vi "Initialize position.vi"(8 "error in (no error)":errorcluster) -> (0 "error out":errorcluster, 3 "Position out":refnum<class "Position.lvclass">)   [LabVIEW 2016, in "Chesslib.lvlib" / "Position.lvclass"]
uses:
  Position.lvclass
  typedef/Color.ctl
  typedef/Square.ctl
  typedef/File.ctl
  typedef/Rank.ctl
  Position.lvclass/Position.ctl
  Chesslib.lvlib
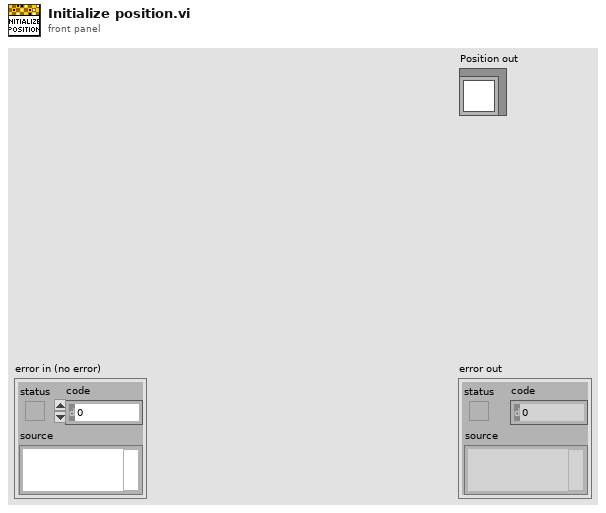
[diagram p1: front panel]
types:
  T1 = typedef "Chesslib.lvlib/Square.ctl" = cluster{"File":T2, "Rank":T3}
  T2 = typedef "Chesslib.lvlib/File.ctl" = enum8{"a", "b", "c", "d", "e", "f", "g", "h"}
  T3 = typedef "Chesslib.lvlib/Rank.ctl" = enum8{"1", "2", "3", "4", "5", "6", "7", "8"}
  T4 = cluster{"White":cluster{"King":bool, "Queen":bool}, "Black":cluster{"King":bool, "Queen":bool}}
  T5 = typedef "Chesslib.lvlib/Color.ctl" = enum16{"White", "Black"}
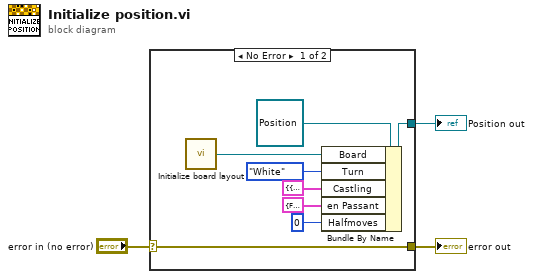
[diagram p0: block diagram]
diagram:
  n1 = case shown="No Error" "error in (no error)" {
    selector: "error in (no error)" -> [w11 w12]
    tunnel: [w11 w12] -> w2
    tunnel: [w9 _] -> w1
    frame No Error {
      n2 = call "Initialize board layout.vi"() -> ("Initialized board"=w4:refnum<class "Board.lvclass">)
      n3 = Bundle By Name(cluster=refnum<class "Position.lvclass"> refnum ("Chesslib.lvlib:Position.lvclass"), "Board"=w4, "Turn"=Color."White", "Castling"=T4 {"White"={"King"=TRUE, "Queen"=TRUE}, "Black"={"King"=TRUE, "Queen"=TRUE}}, "en Passant"=cluster{"Allowed":bool, "Square":T1} {"Allowed"=FALSE, "Square"={"File"=enum."a", "Rank"=enum."1"}}, "Halfmoves"=u8 0) -> (w9:refnum<class "Position.lvclass">)
    }
    frame Error {
    }
  }
  "error out" <- w2
  "Position out" <- w1
